vi "check HOLD and resend.vi"(8 "error in":errorcluster) -> (0 "error out":errorcluster)   [LabVIEW 2016, in "Instrument.OxfordVRM.lvclass"]
uses:
  Instrument.OxfordVRM.lvclass
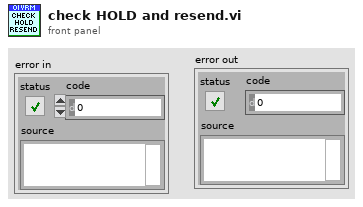
[diagram p1: front panel]
types:
  T1 = typedef "Instrument.OxfordVRM.lvclass/Actions.ctl" = cluster{"Hold":bool, "Clamp":bool, "To Set":bool, "To Zero":bool, "Send to IPS":bool, "PS Heat":bool, "Lambda":bool}
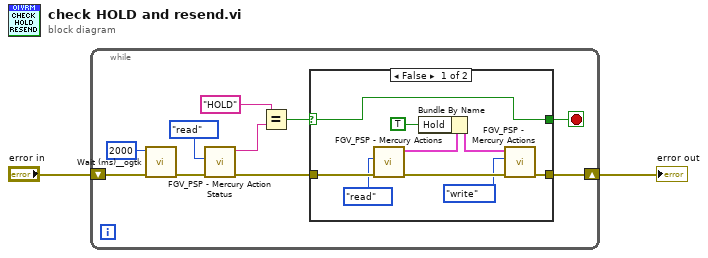
[diagram p0: block diagram]
diagram:
  n1 = while {
    shift-right: [w8] -> w1
    shift-left: "error in" -> [w7]
    stop <- w4 stop-if-true
    n2 = call <userlib>:"Wait (ms)__ogtk.vi"("error in (no error)"=w7, "milliseconds to wait"=u32 2000) -> ("error out"=w6:errorcluster)  [unwired: 8 in, 1 out]
    n3 = call "FGV_PSP - Mercury Action Status.vi"("error in"=w6, "Function"=enum16{"write", "read"}."read") -> ("error out"=w9:errorcluster, "Mercury Status 2"=w3:string)  [unwired: 4 in]
    n4 = Equal?(x="HOLD", y=w3) -> (x = y?=w10:bool)
    n5 = case shown="False" w10 {
      selector: w10 -> [w13 w21]
      tunnel: [w13 w21] -> w4
      tunnel: w9 -> [w19 w22]
      tunnel: [w18 w22] -> w8
      frame False {
        n6 = call "FGV_PSP - Mercury Actions.vi"("error in"=w19, "Function"=enum16{"write", "read"}."read") -> ("Actions"=w15:T1)  [unwired: 4 in, 1 out]
        n7 = Bundle By Name(cluster=w15, "Hold"=TRUE ("Send to IPS")) -> (w14:T1)
        n8 = call "FGV_PSP - Mercury Actions.vi"("error in"=w19, "Function"=enum16{"write", "read"}."write", "Actions"=w14) -> ("error out"=w18:errorcluster)  [unwired: 3 in, 1 out]
      }
      frame True {
      }
    }
  }
  "error out" <- w1
